vi "Add Report Entry.vi"(0 "reference in":refnum<class "Reporter.lvclass">, 2 "comment":string, 3 "step_index":u32, 5 "error in (no error)":errorcluster) -> (14 "reference out":refnum<class "Reporter.lvclass">, 19 "error out":errorcluster)   [LabVIEW 2018, in "Reporter.lvclass"]
uses:
  Reporter.lvclass
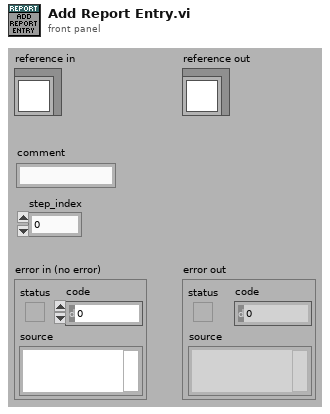
[diagram p1: front panel]
types:
  T1 = typedef "Reporter.lvclass/ObjectAttributes.ctl" = cluster{"LCR":refnum<class "BKP-891 LCR Meter.lvclass">, "PSU":refnum<class "BKP-911x Power Supply.lvclass">, "NI-DAQmx":refnum<class "NI-DAQmx.lvclass">, "Signal List":T2[], "Latest Values":dbl[], "All Latest Values":dbl[], "All Signal List":T2[], "Report Directory":path, "Report File Ref":refnum<file>}
  T2 = typedef "IO Signal List.ctl" = enum16{"Timestamp", "PSU_FB_U_VDC", "PSU_FB_I_AMP", "PSU_FB_W_WATT", "PSU_CMD_U_VDC", "PSU_CMD_I_AMP", "PSU_CMD_OUTPUT", "LCR_PRIMARY", "LCR_SECONDARY", "UV_R_Ohm", "UW_R_Ohm", "VW_R_Ohm", "UV_L_H", "UW_L_H", "VW_L_H", "U_U_VDC", "V_U_VDC", "W_U_VDC", "U_I_AMP", "V_I_AMP", "W_I_AMP", "PWM_CMD_DC_%", "PWM_CMD_VDC", "PWM_CMD_Hz", "PWM_FB_DC_%", "PWM_FB_VDC", "PWM_FB_Hz", "DO_RELAY_U_LCR_A", "DO_RELAY_V_LCR_A", "DO_RELAY_V_LCR_B", "DO_RELAY_W_LCR_B", "DIFF_UV_UW_L_H", "DIFF_UV_VW_L_H", "DIFF_UW_VW_L_H", "DIFF_UV_UW_R_Ohm", "DIFF_UV_VW_R_Ohm", "DIFF_UW_VW_R_Ohm", "DIFF_UV_U_VDC", "DIFF_UW_U_VDC", "DIFF_VW_U_VDC"}
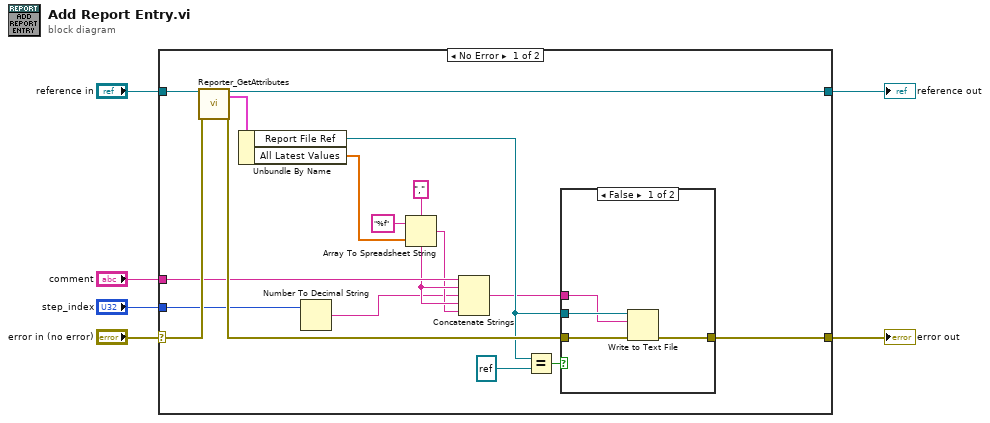
[diagram p0: block diagram]
diagram:
  n1 = case shown="No Error" "error in (no error)" {
    selector: "error in (no error)" -> [w23 w30]
    tunnel: [w13 w30] -> w5
    tunnel: [w20 w29] -> w3
    tunnel: "reference in" -> [w21 w29]
    tunnel: "comment" -> [w12 _]
    tunnel: "step_index" -> [w8 _]
    frame No Error {
      w11 = "," ("delimiter (Tab)")
      n2 = call "Reporter_GetAttributes.vi"("reference in"=w21, "error in (no error)"=w23) -> ("reference out"=w20:refnum<class "Reporter.lvclass">, "Data"=w22:T1, "error out"=w19:errorcluster)  [unwired: 14 in, 1 out]
      n3 = Unbundle By Name(w22) -> ("Report File Ref"=w16:refnum<file>, "All Latest Values"=w15:dbl[])
      n4 = Number To Decimal String(number=w8) -> (decimal integer string=w7:string)  [unwired: 1 in]
      n5 = Array To Spreadsheet String(delimiter (Tab)=w11, array=w15, 3:"%f" ("format string")) -> (spreadsheet string=w10:string)
      n6 = Concatenate Strings(w12, w11, w7, w11, w10) -> (w9:string)
      n7 = Equal?(x=w16, y=refnum<file> refnum) -> (x = y?=w18:bool)
      n8 = case shown="False" w18 {
        tunnel: w19 -> [w27 w28]
        tunnel: w16 -> [w26 _]
        tunnel: [w25 w28] -> w13
        tunnel: w9 -> [w24 _]
        frame False {
          n9 = Write to Text File(file (use dialog)=w26, text=w24, error in=w27) -> (error out=w25:errorcluster)  [unwired: 1 in, 2 out]
        }
        frame True {
        }
      }
    }
    frame Error {
    }
  }
  "error out" <- w5
  "reference out" <- w3
